vi "Hitrap_DiagnosticBox.get move status.vi"(0 "i ref in":refnum<vi>, 2 "Axis":i32, 5 "error in (no error)":errorcluster) -> (14 "i ref out":refnum<vi>, 16 "Moving":bool=TRUE, 17 "Error":bool, 19 "error out":errorcluster)   [LabVIEW 2014, in "Hitrap_DiagnosticBox.lvlib"]
doc: "Get the status information from the motorbase attributes. This VI checks if the step motor is moving or has errors.\n\nThis VI is used in the VI \"Wait\"."
uses:
  Hitrap_DiagnosticBox.lvlib
  CSCore/CSApplicationBaseClasses/MotorBase/MotorBase.statusType.ctl
  CSCore/CSApplicationBaseClasses/MotorBase/MotorBase.lvlib
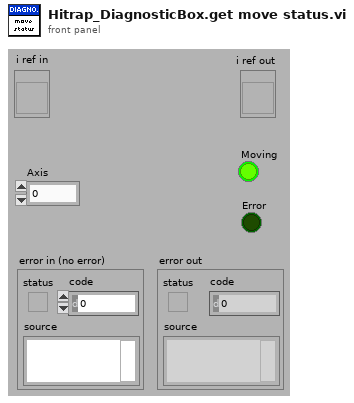
[diagram p1: front panel]
types:
  T1 = typedef "MotorBase.lvlib/MotorBase.statusType.ctl" = u32
  T2 = typedef "MotorBase.lvlib/MotorBase.i attribute.ctl" = cluster{"defaultAxisIndex":i32, "logicalName":string[], "nOfAxes":i32, "physicalName":string[], "scaling":dbl[], "units":string[], "defaulAxisIndexID":i32, "logicalNameID":i32, "nOfAxesID":i32, "physicalNameID":i32, "unitID":i32, "actValues":T3, "nomValues":T3}
  T3 = typedef "MotorBase.lvlib/MotorBase.parameters.ctl" = cluster{"services":cluster{"onOff":bool[], "startVelocity":dbl[], "stopVelocity":dbl[], "acceleration":dbl[], "rangeMin":dbl[], "rangeMax":dbl[], "status":T1[], "position":dbl[]}, "serviceIDs":cluster{"onOffID":i32, "startVelocityID":i32, "stopVelocityID":i32, "accelerationID":i32, "rangeMinID":i32, "rangeMaxID":i32, "statusID":i32, "positionID":i32}}
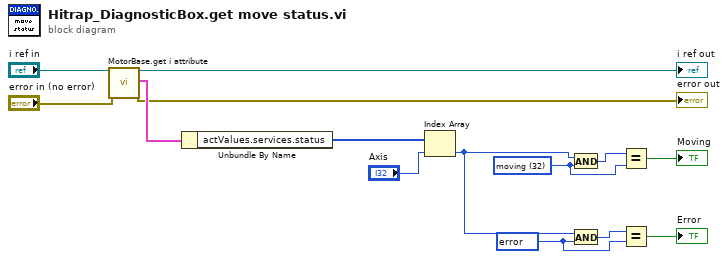
[diagram p0: block diagram]
diagram:
  w1 = T1 4096 items=["motorEnabled"=1, "negativeLimitSwitchActive"=2, "positiveLimitSwitchActive"=4, "limitSwitchesEnabled"=8, "limitSwitchesAreNormallyClosed"=16, "moving"=32, "referenced"=64, "inPosition"=128, "reserved2"=256, "reserved3"=512, "reserved4"=1024, "reserved5"=2048, "error"=4096, "reserved6"=8192, "reserved7"=16384, "reserved8"=32768, "user defined1"=65536, "user defined2"=131072, "user defined3"=262144, "user defined4"=524288, "user defined5"=1048576, "user defined6"=2097152, "user defined7"=4194304, "user defined8"=8388608, "user defined9"=16777216, "user defined10"=33554432, "user defined11"=67108864, "user defined12"=134217728, "user defined13"=268435456, "user defined14"=536870912, "user defined15"=1073741824, "user defined16"=2147483648] ("y")
  w7 = T1 32 items=["motorEnabled"=1, "negativeLimitSwitchActive"=2, "positiveLimitSwitchActive"=4, "limitSwitchesEnabled"=8, "limitSwitchesAreNormallyClosed"=16, "moving"=32, "referenced"=64, "inPosition"=128, "reserved2"=256, "reserved3"=512, "reserved4"=1024, "reserved5"=2048, "error"=4096, "reserved6"=8192, "reserved7"=16384, "reserved8"=32768, "user defined1"=65536, "user defined2"=131072, "user defined3"=262144, "user defined4"=524288, "user defined5"=1048576, "user defined6"=2097152, "user defined7"=4194304, "user defined8"=8388608, "user defined9"=16777216, "user defined10"=33554432, "user defined11"=67108864, "user defined12"=134217728, "user defined13"=268435456, "user defined14"=536870912, "user defined15"=1073741824, "user defined16"=2147483648] ("y")
  n1 = call "MotorBase.get i attribute.vi"("i ref in"="i ref in", "error in (no error)"="error in (no error)") -> ("i ref out"=→"i ref out":refnum<vi>, "i attribute"=w11:T2, "error out"=→"error out":errorcluster)  [unwired: 15 in]
  n2 = Unbundle By Name(w11) -> ("actValues.services.status"=w10:T1[])
  n3 = Index Array(array=w10, index="Axis") -> (element=w6:T1)
  n4 = And(x=w6, y=w7) -> (x .and. y?=w8:T1)
  n5 = And(x=w6, y=w1) -> (x .and. y?=w2:T1)
  n6 = Equal?(x=w8, y=w7) -> (x = y?=→"Moving":bool)
  n7 = Equal?(x=w2, y=w1) -> (x = y?=→"Error":bool)
